vi "JoyIF.vi"(11 "Numeric":dbl) -> (0 "down":bool, 1 "up":bool)   [LabVIEW 2019]
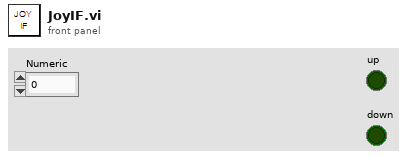
[diagram p1: front panel]
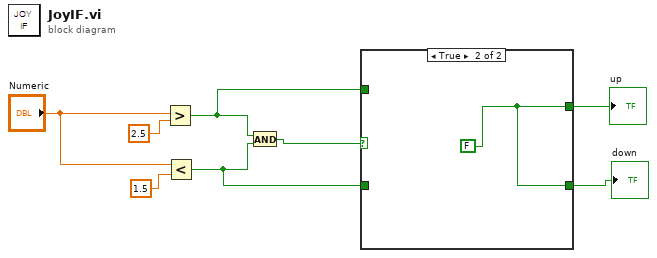
[diagram p0: block diagram]
diagram:
  n1 = Greater?(x="Numeric", y=2.5) -> (0:w4:bool)
  n2 = Less?(x="Numeric", y=1.5) -> (x < y?=w3:bool)
  n3 = And(x=w4, y=w3) -> (x .and. y?=w5:bool)
  n4 = case shown="True" w5 {
    tunnel: w4 -> [w10 _]
    tunnel: w3 -> [w9 _]
    tunnel: [w10 w11] -> w2
    tunnel: [w9 w11] -> w1
    frame False {
    }
    frame True {
      w11 = FALSE
    }
  }
  "down" <- w1
  "up" <- w2
